vi "Parse Parameter.vi"(10 "Parameter":string, 11 "Request.Headers in":variant) -> (3 "Request.Headers out":variant)   [LabVIEW 2023, in "Request.lvclass"]
uses:
  Request.lvclass
  <vilib>/Utility/error.llb/Trim Whitespace One-Sided.vi
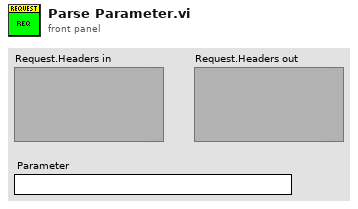
[diagram p1: front panel]
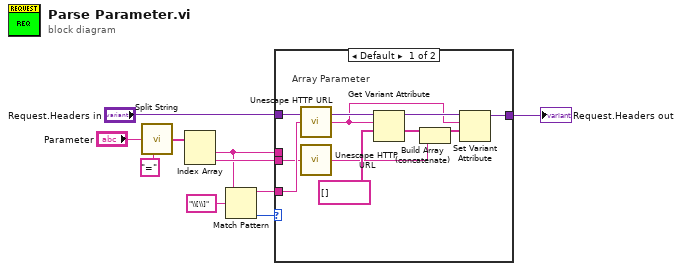
[diagram p0: block diagram]
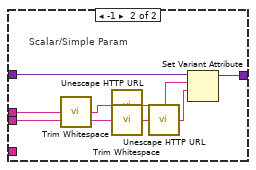
[diagram p2: hidden frame]
diagram:
  n1 = call "Split String.vi"("String"="Parameter", "Delimiter"="=") -> ("Elements"=w9:string[])  [unwired: 7 in]
  n2 = Index Array(array=w9) -> (element #1=w4:string, element #2=w10:string)  [unwired: 2 in]
  n3 = Match Pattern(string=w4, regular expression="\\[\\]") -> (before substring=w1:string, offset past match=w2:i32)  [unwired: 1 in, 2 out]
  n4 = case shown="Default" w2 {
    tunnel: w10 -> [w18 w24]
    tunnel: [w14 w23] -> w8
    tunnel: "Request.Headers in" -> [w20 w22]
    tunnel: w4 -> [_ w21]
    tunnel: w1 -> [w19 _]
    frame Default {
      # "Array Parameter"
      n5 = call "Unescape HTTP URL.vi"("escaped string in"=w19) -> ("unescaped string out"=w11:string)
      n6 = call "Unescape HTTP URL.vi"("escaped string in"=w18) -> ("unescaped string out"=w15:string)
      n7 = Get Variant Attribute(Variant=w20, name=w11, default value (empty Variant)=string[] []) -> (duplicate Variant=w13:variant, value=w16:string[])  [unwired: 1 in, 2 out]
      n8 = Build Array (concatenate)(w16, w15) -> (w12:string[])
      n9 = Set Variant Attribute(Variant=w13, name=w11, value=w12) -> (Variant out=w14:variant)  [unwired: 1 in, 2 out]
    }
    frame -1 {
      # "Scalar/Simple Param"
      n10 = call <vilib>:"Trim Whitespace.vi"("string"=w21) -> ("trimmed string"=w26:string)  [unwired: 1 in]
      n11 = call "Unescape HTTP URL.vi"("escaped string in"=w26) -> ("unescaped string out"=w27:string)
      n12 = call <vilib>:"Trim Whitespace.vi"("string"=w24) -> ("trimmed string"=w25:string)  [unwired: 1 in]
      n13 = call "Unescape HTTP URL.vi"("escaped string in"=w25) -> ("unescaped string out"=w28:string)
      n14 = Set Variant Attribute(Variant=w22, name=w27, value=w28) -> (Variant out=w23:variant)  [unwired: 1 in, 2 out]
    }
  }
  "Request.Headers out" <- w8
